vi "Get-processing-buffer-element.vi"(8 "error in (no error)":errorcluster, 10 "Index":i32, 11 "Buffers in":refnum<class "CV-Buffers.lvclass">) -> (0 "error out":errorcluster, 2 "Element ref":T1[](array[typedef]), 3 "Buffers out":refnum<class "CV-Buffers.lvclass">)   [LabVIEW 2013, in "CameraVision.lvlib" / "CV-Buffers.lvclass"]
uses:
  CV-Buffers.lvclass
  <vilib>/vision/Image Controls.llb/IMAQ Image.ctl
  CV-Buffers.lvclass/CV-Buffers.ctl
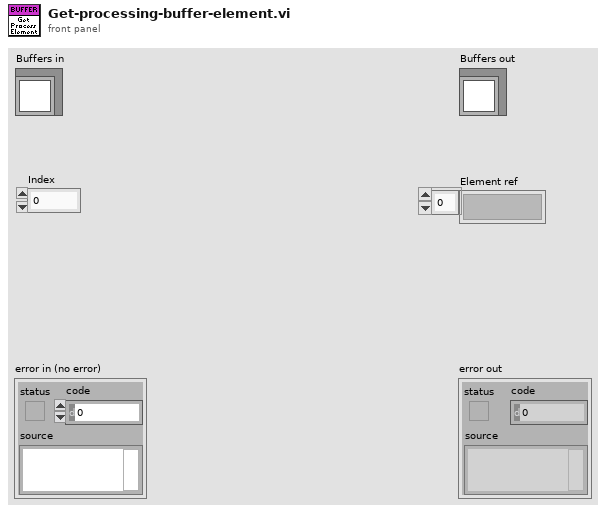
[diagram p1: front panel]
types:
  T1 = typedef "IMAQ Image.ctl" = refnum<image>
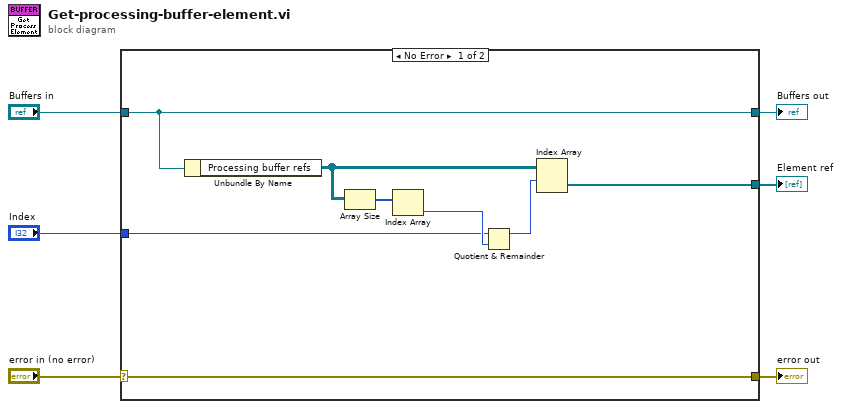
[diagram p0: block diagram]
diagram:
  n1 = case shown="No Error" "error in (no error)" {
    selector: "error in (no error)" -> [w8 w16]
    tunnel: [w8 w16] -> w5
    tunnel: [w14 w15] -> w3
    tunnel: "Buffers in" -> [w14 w15]
    tunnel: "Index" -> [w11 _]
    tunnel: [w7 _] -> w1
    frame No Error {
      n2 = Unbundle By Name(w14) -> ("Processing buffer refs"=w10:T1[][])
      n3 = Array Size(array=w10) -> (size(s)=w13:i32[])
      n4 = Index Array(array=w13) -> (element=w12:i32)  [unwired: 1 in]
      n5 = Quotient & Remainder(x=w11, y=w12) -> (x-y*floor(x/y)=w9:i32)  [unwired: 1 out]
      n6 = Index Array(array=w10, index (row)=w9) -> (element=w7:T1[])  [unwired: 1 in]
    }
    frame Error {
    }
  }
  "error out" <- w5
  "Buffers out" <- w3
  "Element ref" <- w1
